vi "Sequence Graph inquiry.vi"(0 "VISA resource name":refnum<visa-resource-name>, 1 "Start":dbl, 3 "Number":dbl, 5 "Channel  (1: CH1)":u16(ring)=1 items=["CH1"=1, "CH2"=2, "CH3"=3, "CH4"=4], 11 "error in (no error)":errorcluster, 13 "Calculate":bool, 14 "Plot":bool) -> (4 "VISA resource name out":refnum<visa-resource-name>, 6 "Graph":dynamicdata(graph), 8 "Table":string[][](table), 15 "error out":errorcluster)   [LabVIEW 2020, in "GPP.lvlib"]
uses:
  GPP.lvlib
  <vilib>/Platform/TimedLoop/XDataNode/timing_clust.ctl
  <vilib>/Platform/TimedLoop/XDataNode/nitl_modes.ctl
  <vilib>/Platform/TimedLoop/XDataNode/wakeup.ctl
  Function/VISA_COMMON.ctl
  <vilib>/Platform/TimedLoop/XDataNode/XDataNode.xnode
  <vilib>/Platform/TimedLoop/XDataNode/XDNodeRunTimeDep.lvlib
panel:
  in  "历史数据 2":dynamicdata[](array[waveform])
  in  "Table 3":string[][](table)
  in  "In":string
  out "CUT HEAD":string
  out "ADD ;":string
  out "CUT ;":string
  out "AFTER CUT":string
  out "CUT LAST":string
  out "Voltege":dbl
  out "Current":dbl
  out "Time":dbl
  out "Group":dbl
  out "Voltage":dbl[](array[numeric])
  out "Current":dbl[](array[numeric])
  out "Time":dbl[](array[numeric])
  out "Group":dbl[](array[numeric])
  out "Stay":string
  in  "历史数据":dynamicdata[](array[waveform])
  in  "Table 2":string[][](table)
  # "(Read data then plot the Graph)"
  # "(Speed of reading depends on your baud rate)"
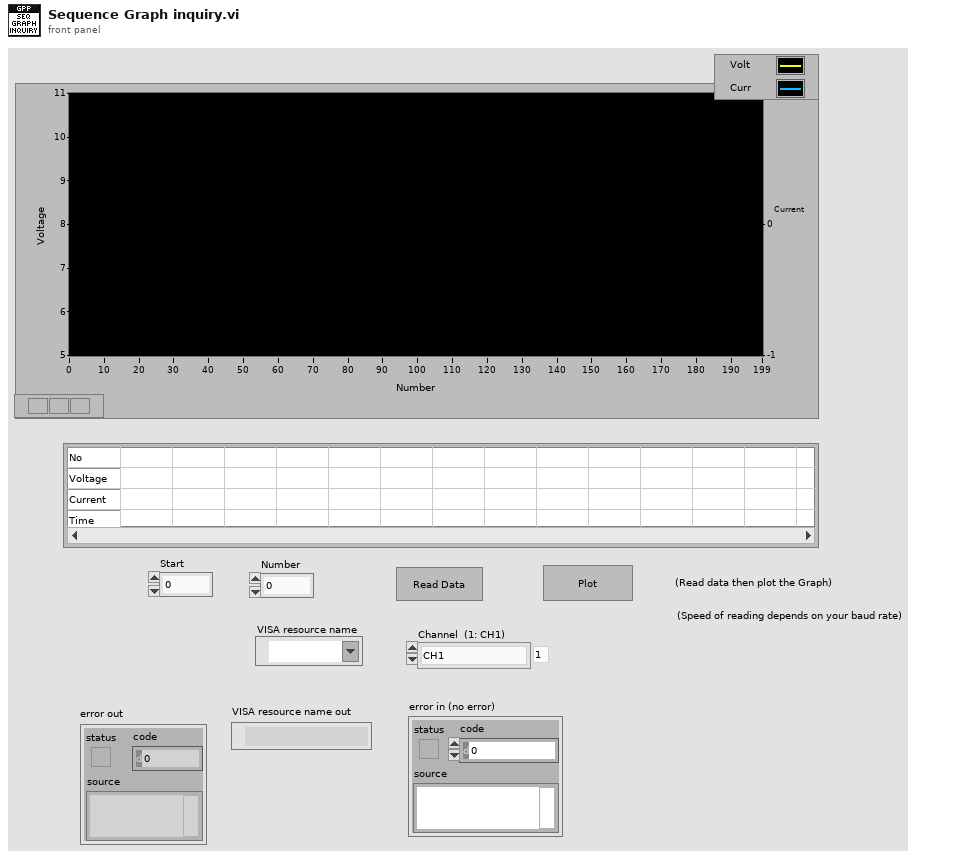
[diagram p1: front panel]
types:
  T1 = typedef "XDNodeRunTimeDep.lvlib/timing_clust.ctl" = cluster{"Expected End [f-1]":u64, "Actual End [f-1]":u64, "Finished Late? [f-1]":bool, "Expected End [i-1]":u64, "Actual End [i-1]":u64, "Finished Late? [i-1]":bool, "Expected Start [i]":u64, "Actual Start [i]":u64, "Expected Start [f]":u64, "Actual Start [f]":u64, "Source Name":string, "Structure Name":string, "Period":i64, "Deadline":i64, "Offset":i64, "Start":i64, "Priority":i32, "Timeout":i32, "Mode":T2, "Wakeup Reason":T3, "Error":errorcluster, "Source Type":string, "Secondary Source Type":string, "Global End Time":u64, "Global Start Time":u64, "Frame Duration":u64, "Iteration Duration":u64, "Assigned CPU":i32, "I/O Scan Engine Mode":u32}
  T2 = typedef "XDNodeRunTimeDep.lvlib/nitl_modes.ctl" = enum32{"No Change", "Process missed periods, maintain original phase", "Discard missed periods, maintain original phase", "Process missed periods, ignore original phase", "Discard missed periods, ignore original phase"}
  T3 = typedef "XDNodeRunTimeDep.lvlib/wakeup.ctl" = enum32{"Normal", "Aborted", "Asynchronous wakeup", "Timing source error", "Timed loop error", "Timeout"}
  T4 = typedef "GPP.lvlib/VISA_COMMON.ctl" = enum16{"Initial", "Write CMD", "Read Result", "Read History", "Close"}
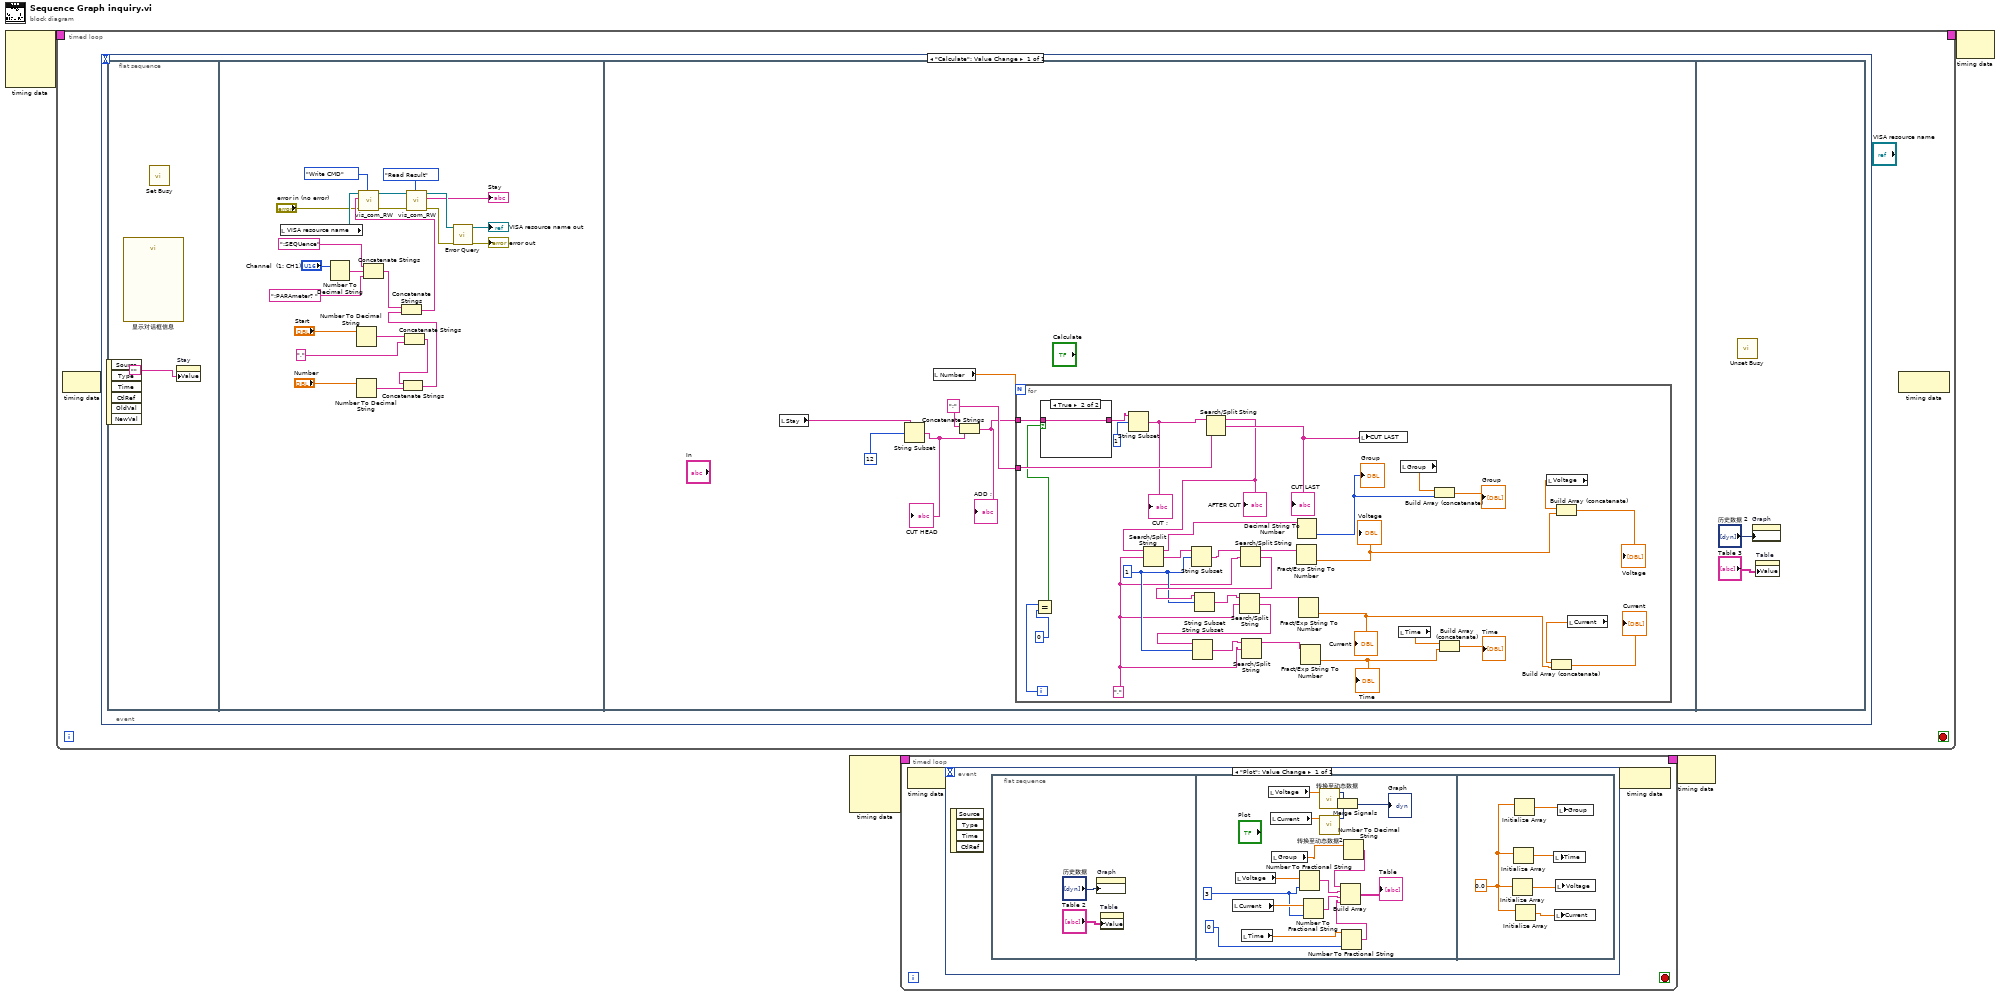
[diagram p0: block diagram]
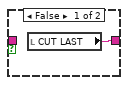
[diagram p2: hidden frame]
diagram:
  n1 = node-c288() -> (w4:T1)  [unwired: 4 in]
  n2 = timed-loop {
    timing: w4 -> [_]
    timing-out: [_] -> w3
    stop <- _ stop-if-true
    n3 = node-c288() -> ()  [unwired: 1 in, 1 out]
    n4 = event shown="[0] \"Calculate\": Value Change" {
      selector: _ -> [_]
      dyn-events: _ -> [_]
      timeout: _ -> [_]
      event "Calculate": Value Change {
        n5 = event-data() -> ()  [unwired: 1 in, 6 out]
        n6 = flat-sequence {
          frame #0 {
            n7 = call "显示对话框信息"() -> ()  [unwired: 10 in, 2 out]
            n8 = call <vilib>:"Set Busy.vi"() -> ()  [unwired: 10 in, 2 out]
            n9 = property on="Stay" class="Str"("Value"="") -> ()  [unwired: 2 in, 2 out]
          }
          frame #1 {
            n10 = local read "VISA resource name"() -> (w29:refnum<visa-resource-name>)
            n11 = Number To Decimal String(number="Channel  (1: CH1)") -> (decimal integer string=w18:string)  [unwired: 1 in]
            n12 = Number To Decimal String(number="Number") -> (decimal integer string=w23:string)  [unwired: 1 in]
            n13 = Number To Decimal String(number="Start") -> (decimal integer string=w26:string)  [unwired: 1 in]
            n14 = Concatenate Strings(":SEQUence", w18, ":PARAmeter? ") -> (w16:string)
            n15 = Concatenate Strings(w26, ",") -> (w24:string)
            n16 = Concatenate Strings(w24, w23) -> (w22:string)
            n17 = Concatenate Strings(w16, w22) -> (w21:string)
            n18 = call "vis_com_RW.vi"("Funciton"=VISA_COMMON."Write CMD", "error in (no error)"="error in (no error)", "CMD String"=w21, "VISA resource in"=w29) -> ("error out"=w9:errorcluster, "VISA resource out"=w10:refnum<visa-resource-name>)  [unwired: 5 in, 1 out]
            n19 = call "vis_com_RW.vi"("Funciton"=VISA_COMMON."Read Result", "error in (no error)"=w9, "VISA resource in"=w10) -> ("error out"=w7:errorcluster, "Result"=→"Stay":string, "VISA resource out"=w8:refnum<visa-resource-name>)  [unwired: 6 in]
            n20 = call "Error Query.vi"("error in (no error)"=w7, "VISA resource name"=w8) -> ("error out"=→"error out":errorcluster, "VISA resource name out"=→"VISA resource name out":refnum<visa-resource-name>)  [unwired: 6 in, 2 out]
          }
          frame #2 {
            w33 = ";"
            n21 = local read "Stay"() -> (w30:string)
            n22 = String Subset(string=w30, offset (0)=12) -> (substring=w34:string)  [unwired: 1 in]
            "CUT HEAD" <- w34
            n23 = local read "Number"() -> (w31:dbl)
            n24 = Concatenate Strings(w33, w34) -> (w32:string)
            "ADD ;" <- w32
            n25 = for {
              N: w31 -> [_]
              tunnel: w33 -> [w69]
              tunnel: w32 -> [w37]
              i -> [w39]
              w59 = 1
              w57 = ","
              n26 = Equal?(x=w39, y=0) -> (x = y?=w38:bool)
              n27 = case shown="True" w38 {
                tunnel: w37 -> [_ w71]
                tunnel: [w70 w71] -> w36
                frame False {
                  n28 = local read "CUT LAST"() -> (w70:string)
                }
                frame True {
                }
              }
              n29 = String Subset(string=w36, offset (0)=1) -> (substring=w68:string)  [unwired: 1 in]
              "CUT ;" <- w68
              n30 = Search/Split String(string=w68, search string/char (-)=w69) -> (substring before match=w65:string, match + rest of string=w66:string)  [unwired: 1 in, 1 out]
              "AFTER CUT" <- w65
              "CUT LAST" <- w66
              n31 = Search/Split String(string=w65, search string/char (-)=w57) -> (substring before match=w53:string, match + rest of string=w64:string)  [unwired: 1 in, 1 out]
              n32 = String Subset(string=w64, offset (0)=w59) -> (substring=w63:string)  [unwired: 1 in]
              n33 = Search/Split String(string=w63, search string/char (-)=w57) -> (substring before match=w56:string, match + rest of string=w62:string)  [unwired: 1 in, 1 out]
              n34 = String Subset(string=w62, offset (0)=w59) -> (substring=w61:string)  [unwired: 1 in]
              n35 = Search/Split String(string=w61, search string/char (-)=w57) -> (substring before match=w55:string, match + rest of string=w60:string)  [unwired: 1 in, 1 out]
              n36 = String Subset(string=w60, offset (0)=w59) -> (substring=w58:string)  [unwired: 1 in]
              n37 = Search/Split String(string=w58, search string/char (-)=w57) -> (substring before match=w54:string)  [unwired: 1 in, 2 out]
              n38 = Fract/Exp String To Number(string=w56) -> (number=w52:dbl)  [unwired: 3 in, 1 out]
              "Voltege" <- w52
              n39 = Decimal String To Number(string=w53) -> (number=w46:i32)  [unwired: 2 in, 1 out]
              "Group" <- w46
              n40 = Fract/Exp String To Number(string=w55) -> (number=w50:dbl)  [unwired: 3 in, 1 out]
              "Current" <- w50
              n41 = Fract/Exp String To Number(string=w54) -> (number=w43:dbl)  [unwired: 3 in, 1 out]
              "Time" <- w43
              n42 = local write "CUT LAST"(w66) -> ()
              n43 = local read "Time"() -> (w42:dbl[])
              n44 = local read "Group"() -> (w45:dbl[])
              n45 = Build Array (concatenate)(w45, w46) -> (→"Group":dbl[])
              n46 = Build Array (concatenate)(w42, w43) -> (→"Time":dbl[])
              n47 = local read "Voltage"() -> (w48:dbl[])
              n48 = Build Array (concatenate)(w48, w52) -> (→"Voltage":dbl[])
              n49 = local read "Current"() -> (w47:dbl[])
              n50 = Build Array (concatenate)(w47, w50) -> (→"Current":dbl[])
            }
          }
          frame #3 {
            n51 = call <vilib>:"Unset Busy.vi"() -> ()  [unwired: 11 in, 1 out]
            n52 = property on="Graph" class="WFChart (strict)"("History Data"="历史数据 2") -> ()  [unwired: 2 in, 2 out]
            n53 = property on="Table" class="Tbl (strict)"("Value"="Table 3") -> ()  [unwired: 2 in, 2 out]
          }
        }
      }
    }
    n54 = node-c288() -> ()  [unwired: 1 in, 1 out]
  }
  n55 = node-c288() -> (w2:T1)  [unwired: 4 in]
  n56 = timed-loop {
    timing: w2 -> [_]
    timing-out: [_] -> w1
    stop <- _ stop-if-true
    n57 = node-c288() -> ()  [unwired: 1 in, 1 out]
    n58 = event shown="[0] \"Plot\": Value Change" {
      selector: _ -> [_]
      dyn-events: _ -> [_]
      timeout: _ -> [_]
      event "Plot": Value Change {
        n59 = event-data() -> ()  [unwired: 1 in, 4 out]
        n60 = flat-sequence {
          frame #0 {
            n61 = property on="Graph" class="WFChart (strict)"("History Data"="历史数据") -> ()  [unwired: 2 in, 2 out]
            n62 = property on="Table" class="Tbl (strict)"("Value"="Table 2") -> ()  [unwired: 2 in, 2 out]
          }
          frame #1 {
            w79 = 3
            n63 = local read "Current"() -> (w84:dbl[])
            n64 = local read "Voltage"() -> (w85:dbl[])
            n65 = local read "Time"() -> (w86:dbl[])
            n66 = local read "Voltage"() -> (w93:dbl[])
            n67 = local read "Current"() -> (w91:dbl[])
            n68 = local read "Group"() -> (w87:dbl[])
            n69 = Number To Fractional String(number=w85, precision (6)=w79) -> (F-format string=w83:string[])  [unwired: 2 in]
            n70 = Number To Fractional String(number=w84, precision (6)=w79) -> (F-format string=w81:string[])  [unwired: 2 in]
            n71 = call "转换至动态数据"("Array"=w93) -> ("Dynamic Data Type"=w92:dynamicdata)  [unwired: 3 in]
            n72 = call "转换至动态数据2"("Array"=w91) -> ("Dynamic Data Type"=w90:dynamicdata)  [unwired: 3 in]
            n73 = Merge Signals(w92, w90) -> (→"Graph":dynamicdata)
            n74 = Number To Fractional String(number=w86, precision (6)=0) -> (F-format string=w80:string[])  [unwired: 2 in]
            n75 = Number To Decimal String(number=w87) -> (decimal integer string=w82:string[])  [unwired: 1 in]
            n76 = Build Array(w82, w83, w81, w80) -> (→"Table":string[][])
          }
          frame #2 {
            w97 = 0.0
            n77 = Initialize Array(w97) -> (w95:dbl[])  [unwired: 1 in]
            n78 = Initialize Array(w97) -> (w96:dbl[])  [unwired: 1 in]
            n79 = Initialize Array(w97) -> (w98:dbl[])  [unwired: 1 in]
            n80 = Initialize Array(w97) -> (w94:dbl[])  [unwired: 1 in]
            n81 = local write "Time"(w96) -> ()
            n82 = local write "Current"(w94) -> ()
            n83 = local write "Voltage"(w95) -> ()
            n84 = local write "Group"(w98) -> ()
          }
        }
      }
    }
    n85 = node-c288() -> ()  [unwired: 1 in, 1 out]
  }
  n86 = node-c288(w1) -> ()  [unwired: 1 out]
  n87 = node-c288(w3) -> ()  [unwired: 1 out]
